vi "Range of w (SubVI).vi"() -> (2 "-pi to pi":dbl[](array[numeric]))   [LabVIEW 2014]
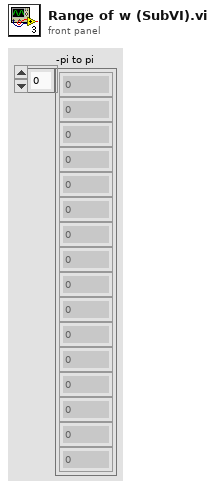
[diagram p1: front panel]
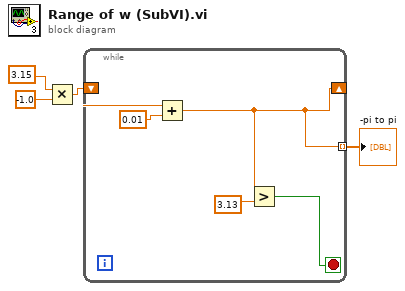
[diagram p0: block diagram]
diagram:
  n1 = Multiply(x=3.15, y=-1.0) -> (x*y=w3:dbl)
  n2 = while {
    shift-right: [w7] -> _
    shift-left: w3 -> [w6]
    tunnel: [w7] -> w1 mode=indexing
    stop <- w9 stop-if-true
    n3 = Add(x=w6, y=0.01) -> (x+y=w7:dbl)
    n4 = Greater?(x=w7, y=3.13) -> (0:w9:bool)
  }
  "-pi to pi" <- w1
